vi "Delays.vi"(0 "sound spd (cm/s)":i32, 2 "rings":dbl[](array[numeric]), 3 "radius":dbl, 4 "DR Inputs":T1 {"Tansducer" items=["F2 40 MHz", "F3 20 MHz"]}) -> (5 "delays":dbl[](array[numeric]) format="%#_3e")   [LabVIEW 2022 SP3]
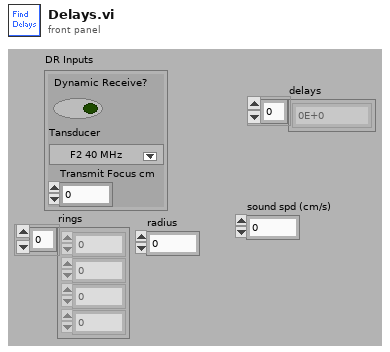
[diagram p1: front panel]
types:
  T1 = cluster{"Dynamic Receive?":bool, "Tansducer":u16, "Transmit Focus cm":dbl}
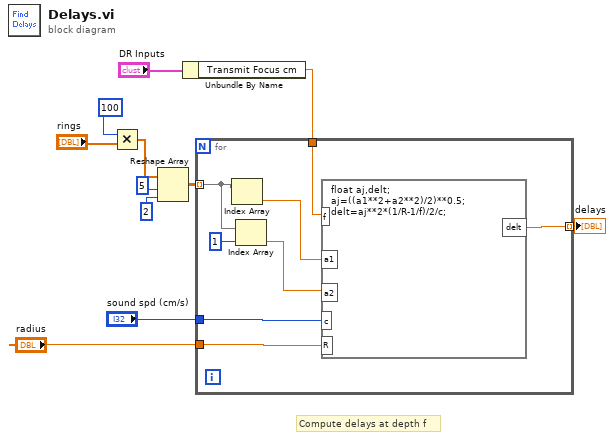
[diagram p0: block diagram]
diagram:
  # "Compute delays at depth f"
  n1 = Multiply(x=100, y="rings") -> (x*y=w4:dbl[])
  n2 = Reshape Array(w4, 5, 2) -> (w10:dbl[][])
  n3 = Unbundle By Name("DR Inputs") -> ("Transmit Focus cm"=w5:dbl)
  n4 = for {
    tunnel: w10 -> [w19] mode=indexing
    tunnel: [w15] -> w7 mode=indexing
    tunnel: w5 -> [w14]
    tunnel: "sound spd (cm/s)" -> [w13]
    tunnel: "radius" -> [w12]
    n5 = Index Array(array=w19) -> (element=w17:dbl)  [unwired: 1 in]
    n6 = Index Array(array=w19, index=1) -> (element=w16:dbl)
    n7 = formula code="float aj,delt;\naj=((a1**2+a2**2)/2)**0.5;\ndelt=aj**2*(1/R-1/f)/2/c;"("R"=w12, "f"=w14, "a1"=w17, "a2"=w16, "c"=w13) -> ("delt"=w15:dbl)
  }
  "delays" <- w7
